vi "WebSocket Write Json.vi"(8 "error in":errorcluster, 9 "timeout ms (5000)":i32=5000, 10 "Websocket Command":T1={"Command"="Encoder", "Data"=""}, 11 "WebSocket Connection in":refnum<k5>) -> (0 "error out":errorcluster, 3 "WebSocket Connection out":refnum<k5>)   [LabVIEW 2018]
uses:
  Data Def/Websocket Command.ctl
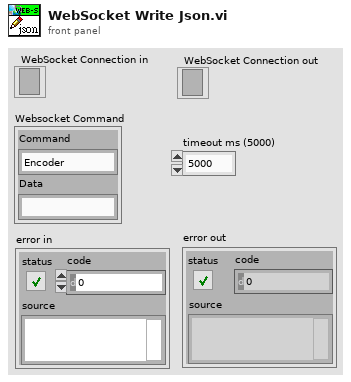
[diagram p1: front panel]
types:
  T1 = typedef "Websocket Command.ctl" = cluster{"Command":string, "Data":string}
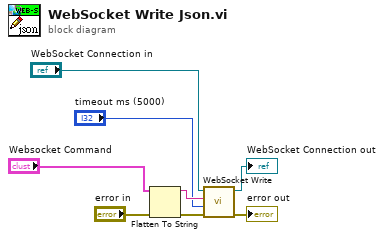
[diagram p0: block diagram]
diagram:
  n1 = Flatten To String(anything="Websocket Command", error in (no error)="error in") -> (data string=w8:string, error out=w7:errorcluster)  [unwired: 2 in, 1 out]
  n2 = call "WebSocket Write.vi"("error in"=w7, "timeout ms (5000)"="timeout ms (5000)", "Data"=w8, "WebSocket Connection in"="WebSocket Connection in") -> ("error out"=→"error out":errorcluster, "WebSocket Connection out"=→"WebSocket Connection out":refnum<k5>)  [unwired: 6 in]
